vi "Legend Palette.vi"(4 "Active Plot":i32, 6 "Control Ref Queue":T4, 9 "Window Bounds":T5, 10 "Multiplot Representation In":T1, 11 "2D Feather.lvclass in":refnum<class "2D Feather.lvclass">) -> (1 "Cancel?":bool, 2 "Multiplot Representation Out":T1, 3 "2D Feather.lvclass out":refnum<class "2D Feather.lvclass">)   [LabVIEW 2020, in "2D Feather.lvclass"]
uses:
  <vilib>/Math Plots/2D Math Plots/2D Feather/2D Feather/2D Feather.lvclass
  e:/builds/penguin/labview/branches/2020/dev/dist/vi.lib/Math Plots/2D Math Plots/2D Plot/2D Plot/2D Plot.lvclass
  <vilib>/Math Plots/2D Math Plots/2D Plot/Action String/2DMathPlot Ctrl Act Queue.ctl
  <vilib>/Math Plots/2D Math Plots/2D Plot/Action String/2DMathPlot Ctrl Act Cluster.ctl
  <vilib>/Math Plots/2D Math Plots/2D Plot/Action String/2DMathPlot State Class.ctl
  <vilib>/Math Plots/2D Math Plots/2D Plot/2D Plot/Typedef/Multiplot Representation.ctl
  <vilib>/Math Plots/2D Math Plots/2D Plot/2D Plot/Typedef/Plot Representation.ctl
  <vilib>/Math Plots/2D Math Plots/2D Plot/2D Plot/Typedef/Range Cluster.ctl
  <vilib>/Utility/miscctls.llb/LVRectTypeDef.ctl
  <vilib>/Math Plots/2D Math Plots/2D Feather/2D Feather/2D Feather.lvclass/2D Feather.ctl
  <vilib>/Math Plots/2D Math Plots/2D Plot/2D Plot/2D Plot.lvclass
panel:
  in  "Tab Control":enum32{"Plot Property", "Input & Output"}(tab)
  in  "Line Width":u16(ring) caption="Line width"
  in  "Line Style":u16(ring) caption="Line style"
  in  "OK":bool
  in  "Cancel":bool
  in  "Feather Size":dbl caption="Feather size"
  in  "Feather Color":u32(colorbox)
  # "Line style"
  # "Line width"
  # "Feather size"
  # "Feather color"
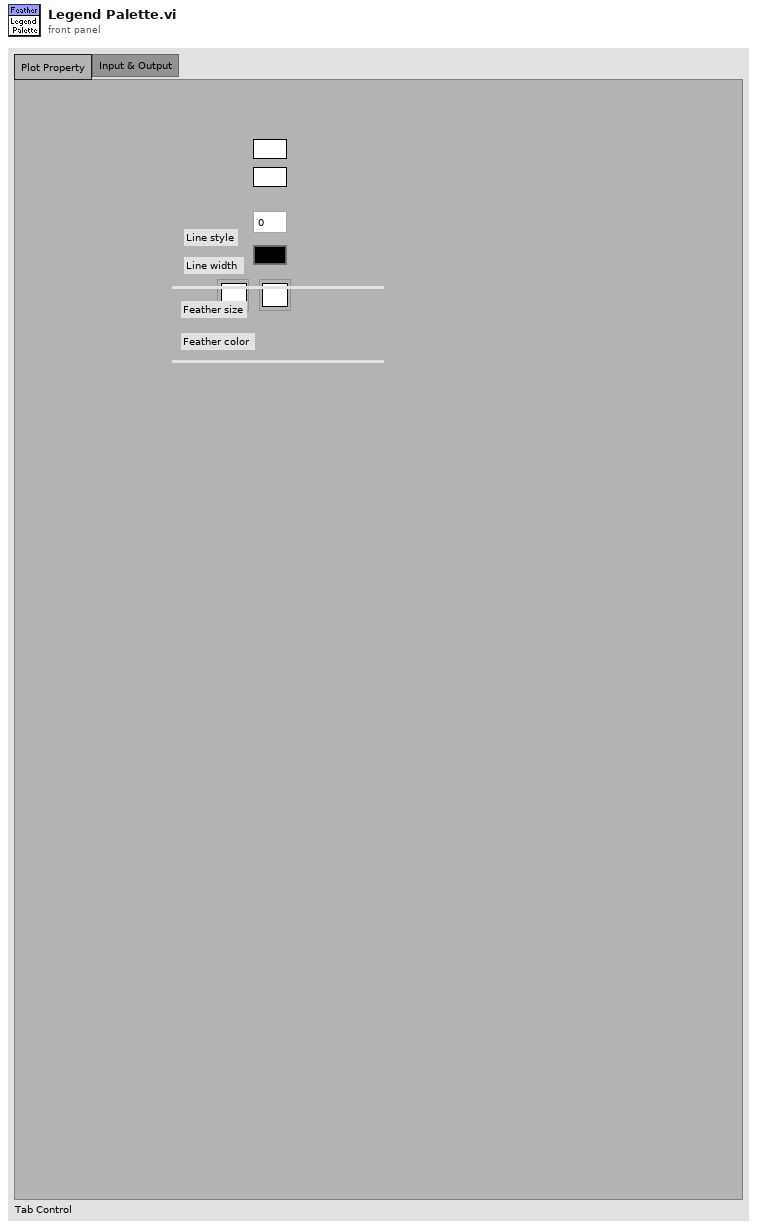
[diagram p1: front panel]
types:
  T1 = typedef "2D Plot.lvclass/Multiplot Representation.ctl" = cluster{"Plot Representation Array":T2[], "Max Range":T3}
  T2 = typedef "2D Plot.lvclass/Plot Representation.ctl" = cluster{"Plot Range":T3, "Vertex Cluster":cluster{"Vertex X Array":dbl[], "Vertex Y Array":dbl[]}, "Base Cluster":cluster{"Base X Array":dbl[], "Base Y Array":dbl[]}}
  T3 = typedef "2D Plot.lvclass/Range Cluster.ctl" = cluster{"X Range":cluster{"Max X":dbl, "Min X":dbl}, "Y Range":cluster{"Max Y":dbl, "Min Y":dbl}}
  T4 = typedef "2DMathPlot Ctrl Act Queue.ctl" = refnum<queue>
  T5 = typedef "LVRectTypeDef.ctl" = cluster{"Left":i16, "Top":i16, "Right":i16, "Bottom":i16}
  T6 = typedef "2DMathPlot Ctrl Act Cluster.ctl" = cluster{"Plot Area Ref":refnum<vi>, "Z Axis Ref":refnum<vi>, "Legend Ref":refnum<vi>, "XControl Ref":refnum<vi>, "Facade Ref":refnum<vi>, "Display State Change Class":T7}
  T7 = typedef "2DMathPlot State Class.ctl" = enum16{"Update All (Undo)", "Update General", "Update Appearance", "Update Format", "Update Scale", "Update Marker", "Update Cursor", "None"}
  T8 = typedef "2D Plot.lvclass/Plot Property Array.ctl" = T9[]
  T9 = typedef "2D Plot.lvclass/Plot Property.ctl" = cluster{"Bar Plot Style":u8, "DigitalLineStyle":u8, "TransitionLocation":u8, "Transition Type":u8, "Fill To":i16, "Fill/Pt. Color":u32, "Label Style":u8, "Line Style":u8, "Line Width":u8, "Plot Color":u32, "Plot Interpolation":u8, "Plot Name":string, "Point Style":u8, "Visible?":bool, "XScaleIdx":u32, "YScaleIdx":u32}
  T10 = typedef "2D Feather.lvclass/2D Feather Property Array.ctl" = T11[]
  T11 = typedef "2D Feather.lvclass/2D Feather Property.ctl" = cluster{"Arrow Size":dbl}
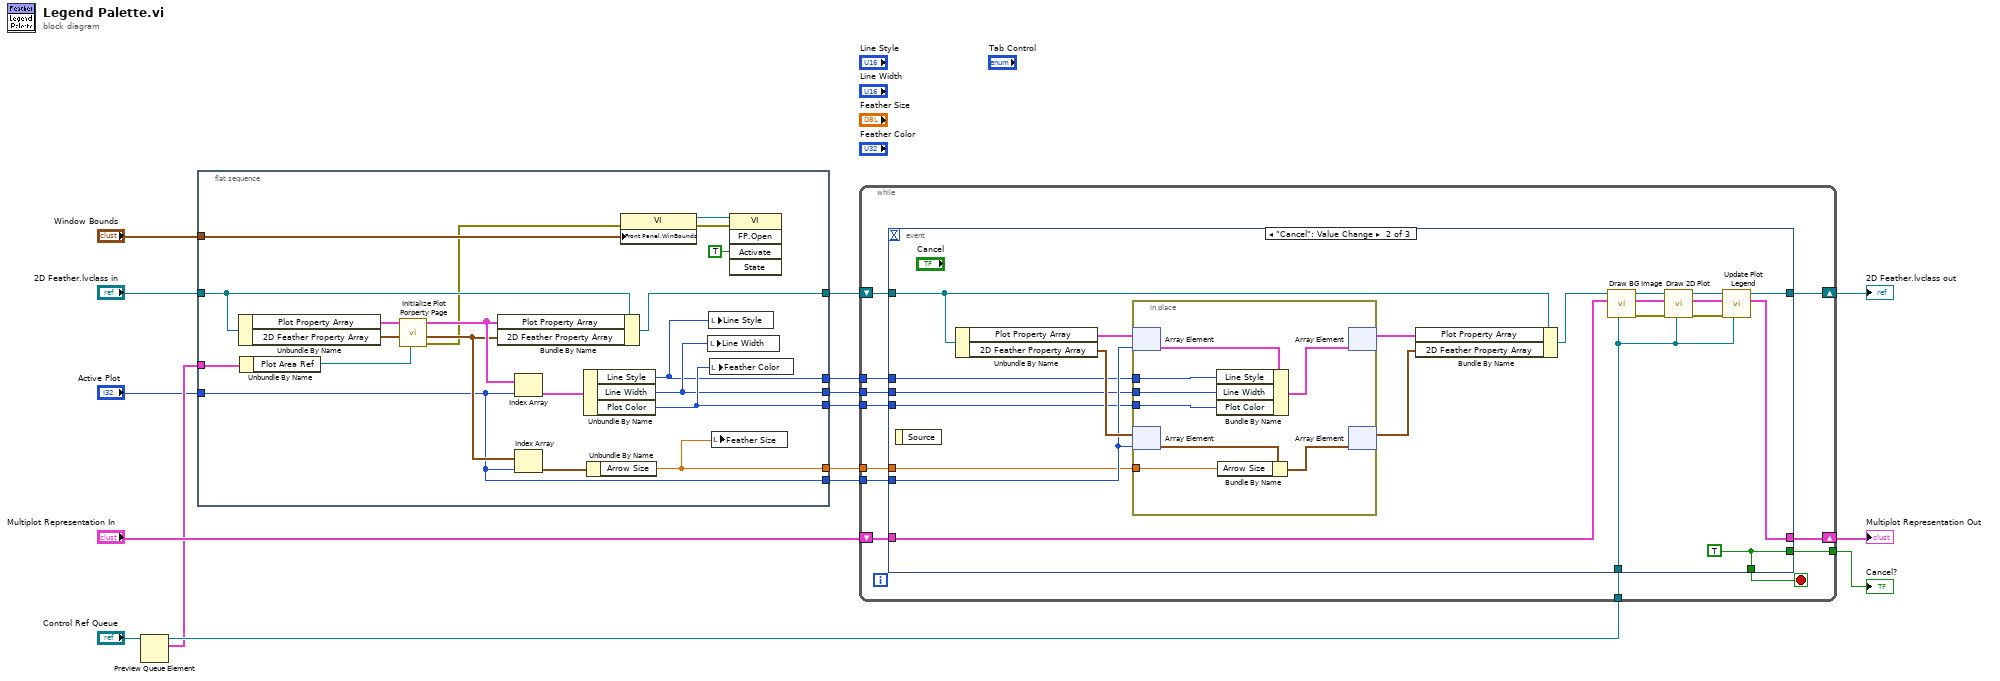
[diagram p0: block diagram]
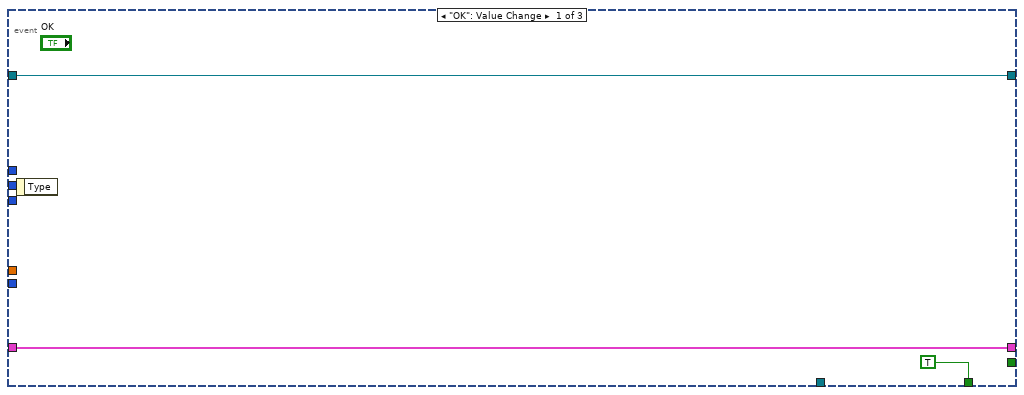
[diagram p2: hidden frame]
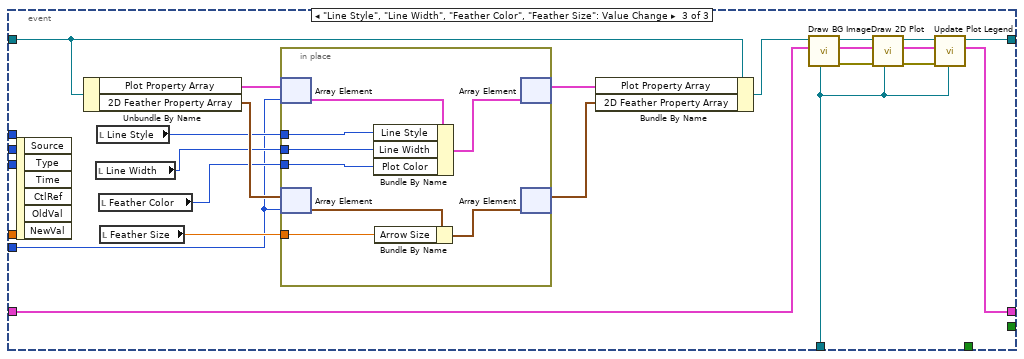
[diagram p3: hidden frame]
diagram:
  n1 = Preview Queue Element(queue="Control Ref Queue") -> (queue out=w10:T4, element=w9:T6)  [unwired: 1 in, 3 out]
  n2 = flat-sequence {
    tunnel: "2D Feather.lvclass in" -> [w29]
    tunnel: [w28] -> w14
    tunnel: [w20] -> w4
    tunnel: w9 -> [w34]
    tunnel: [w33] -> w8
    tunnel: [w32] -> w7
    tunnel: [w31] -> w6
    tunnel: [w30] -> w5
    tunnel: "Window Bounds" -> [w22]
    tunnel: "Active Plot" -> [w20]
    frame #0 {
      n3 = Unbundle By Name(w29) -> ("Plot Property Array"=w27:T8, "2D Feather Property Array"=w23:T10)
      n4 = Unbundle By Name(w34) -> ("Plot Area Ref"=w25:refnum<vi>)
      n5 = call <vilib>:"Initialize Plot Porperty Page.vi"("Plot Area Ref"=w25, "2D Featherr Array In"=w23, "Plot Property Array In"=w27) -> ("error out"=w21:errorcluster, "2D Feather Array Out"=w24:T10, "Plot Property Array Out"=w26:T8)  [unwired: 2 in, 4 out]
      n6 = Bundle By Name(cluster=w29, "Plot Property Array"=w26, "2D Feather Property Array"=w24) -> (w28:refnum<class "2D Feather.lvclass">)
      n7 = Index Array(array=w26, index=w20) -> (element=w36:T9)
      n8 = Index Array(array=w24, index=w20) -> (element=w35:T11)
      n9 = Unbundle By Name(w36) -> ("Line Style"=w30:u8, "Line Width"=w31:u8, "Plot Color"=w32:u32)
      n10 = Unbundle By Name(w35) -> ("Arrow Size"=w33:dbl)
      n11 = property class="VI"(error in=w21, "Front Panel.WinBounds"=w22) -> (reference out=w19:refnum<vi>, error out=w18:errorcluster)  [unwired: 1 in]
      n12 = local write "Line Width"(w31) -> ()
      n13 = local write "Line Style"(w30) -> ()
      n14 = local write "Feather Color"(w32) -> ()
      n15 = local write "Feather Size"(w33) -> ()
      n16 = invoke class="VI" method="FP.Open"(reference=w19, error in=w18, "Activate"=TRUE ("Activate?")) -> ()  [unwired: 2 in, 5 out]
    }
  }
  n17 = while {
    shift-right: [w47] -> w16
    shift-left: w14 -> [w48]
    shift-right: [w45] -> w12
    shift-left: "Multiplot Representation In" -> [w46]
    tunnel: w10 -> [w44]
    tunnel: w4 -> [w43]
    tunnel: w8 -> [w41]
    tunnel: w7 -> [w40]
    tunnel: w6 -> [w39]
    tunnel: w5 -> [w38]
    tunnel: [w37] -> w3
    stop <- w42 stop-if-true
    n18 = event shown="[1] \"Cancel\": Value Change" {
      selector: _ -> [_ _ _]
      dyn-events: _ -> [_ _ _]
      timeout: _ -> [_ _ _]
      tunnel: w48 -> [w51 w68 w100]
      tunnel: [w51 w61 w90] -> w47
      tunnel: w46 -> [w50 w67 w92]
      tunnel: [w50 w60 w89] -> w45
      tunnel: w44 -> [_ w53 w82]
      tunnel: w43 -> [_ w66 w91]
      tunnel: [TRUE w52 _] -> w42
      tunnel: w41 -> [_ w65 _]
      tunnel: w40 -> [_ w64 _]
      tunnel: w39 -> [_ w63 _]
      tunnel: w38 -> [_ w62 _]
      tunnel: [_ w52 _] -> w37
      event "OK": Value Change {
        n19 = event-data() -> ()  [unwired: 2 out]
      }
      event "Cancel": Value Change {
        w52 = TRUE
        n20 = event-data() -> ()  [unwired: 2 out]
        n21 = Unbundle By Name(w68) -> ("Plot Property Array"=w73:T8, "2D Feather Property Array"=w72:T10)
        n22 = in-place {
          in-place-border: w65 -> [w77]
          in-place-border: w62 -> [w76]
          in-place-border: w63 -> [w75]
          in-place-border: w64 -> [w74]
          n23 = in-place-array #1(w73, w66) -> (w81:T9)
          n24 = in-place-array #2(w72, w66) -> (w80:T11)
          n25 = Bundle By Name(cluster=w81, "Line Style"=w76, "Line Width"=w75, "Plot Color"=w74) -> (w78:T9)
          n26 = Bundle By Name(cluster=w80, "Arrow Size"=w77) -> (w79:T11)
          n27 = in-place-array #1(w78) -> (w71:T8)  [unwired: 1 out]
          n28 = in-place-array #2(w79) -> (w70:T10)  [unwired: 1 out]
        }
        n29 = Bundle By Name(cluster=w68, "Plot Property Array"=w71, "2D Feather Property Array"=w70) -> (w69:refnum<class "2D Feather.lvclass">)
        n30 = call-dynamic "Draw BG Image.vi"("Control Ref Queue"=w53, "Multiplot Representation In"=w67, "2D Feather.lvclass in"=w69) -> ("error out"=w59:errorcluster, "Multiplot Representation Out"=w58:T1, "2D Feather.lvclass out"=w57:refnum<class "2D Feather.lvclass">)  [unwired: 1 in, 5 out]
        n31 = call-dynamic "Draw 2D Plot.vi"("Control Ref Queue"=w53, "error in (no error)"=w59, "Multiplot Representation In"=w58, "2D Feather.lvclass in"=w57) -> ("error out"=w54:errorcluster, "Multiplot Representation Out"=w55:T1, "2D Feather.lvclass out"=w56:refnum<class "2D Feather.lvclass">)  [unwired: 5 out]
        n32 = call <vilib>:"Update Plot Legend.vi"("Control Ref Queue"=w53, "error in (no error)"=w54, "Multiplot Representation In"=w55, "2D Plot in"=w56) -> ("Multiplot Representation Out"=w60:T1, "2D Plot out"=w61:refnum<class "2D Feather.lvclass">)  [unwired: 6 out]
      }
      event "Line Style", "Line Width", "Feather Color", "Feather Size": Value Change {
        n33 = event-data() -> ()  [unwired: 7 out]
        n34 = Unbundle By Name(w100) -> ("Plot Property Array"=w102:T8, "2D Feather Property Array"=w101:T10)
        n35 = local read "Line Width"() -> (w95:u16)
        n36 = local read "Line Style"() -> (w96:u16)
        n37 = local read "Feather Color"() -> (w94:u32)
        n38 = local read "Feather Size"() -> (w97:dbl)
        n39 = in-place {
          in-place-border: w97 -> [w106]
          in-place-border: w96 -> [w105]
          in-place-border: w95 -> [w104]
          in-place-border: w94 -> [w103]
          n40 = in-place-array #3(w102, w91) -> (w110:T9)
          n41 = in-place-array #4(w101, w91) -> (w109:T11)
          n42 = Bundle By Name(cluster=w110, "Line Style"=w105, "Line Width"=w104, "Plot Color"=w103) -> (w107:T9)
          n43 = Bundle By Name(cluster=w109, "Arrow Size"=w106) -> (w108:T11)
          n44 = in-place-array #3(w107) -> (w99:T8)  [unwired: 1 out]
          n45 = in-place-array #4(w108) -> (w98:T10)  [unwired: 1 out]
        }
        n46 = Bundle By Name(cluster=w100, "Plot Property Array"=w99, "2D Feather Property Array"=w98) -> (w93:refnum<class "2D Feather.lvclass">)
        n47 = call-dynamic "Draw BG Image.vi"("Control Ref Queue"=w82, "Multiplot Representation In"=w92, "2D Feather.lvclass in"=w93) -> ("error out"=w88:errorcluster, "Multiplot Representation Out"=w87:T1, "2D Feather.lvclass out"=w86:refnum<class "2D Feather.lvclass">)  [unwired: 1 in, 5 out]
        n48 = call-dynamic "Draw 2D Plot.vi"("Control Ref Queue"=w82, "error in (no error)"=w88, "Multiplot Representation In"=w87, "2D Feather.lvclass in"=w86) -> ("error out"=w83:errorcluster, "Multiplot Representation Out"=w84:T1, "2D Feather.lvclass out"=w85:refnum<class "2D Feather.lvclass">)  [unwired: 5 out]
        n49 = call <vilib>:"Update Plot Legend.vi"("Control Ref Queue"=w82, "error in (no error)"=w83, "Multiplot Representation In"=w84, "2D Plot in"=w85) -> ("Multiplot Representation Out"=w89:T1, "2D Plot out"=w90:refnum<class "2D Feather.lvclass">)  [unwired: 6 out]
      }
    }
  }
  "2D Feather.lvclass out" <- w16
  "Multiplot Representation Out" <- w12
  "Cancel?" <- w3
